vi "SaveDown.vi"(9 "DataPile":T1(array[cluster]), 10 "Analytes":string[](array[string])) -> ()   [LabVIEW 2024]
panel:
  in  "t0":timestamp
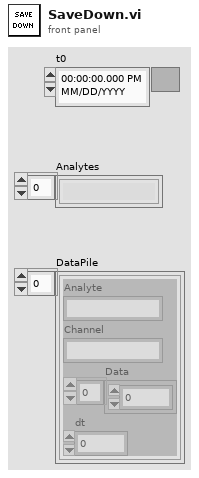
[diagram p1: front panel]
types:
  T1 = cluster{"Analyte":string, "Channel":string, "Data":dbl[], "dt":dbl}[]
  T2 = enum16{"open", "open or create", "create or replace", "create", "open (read-only)"}
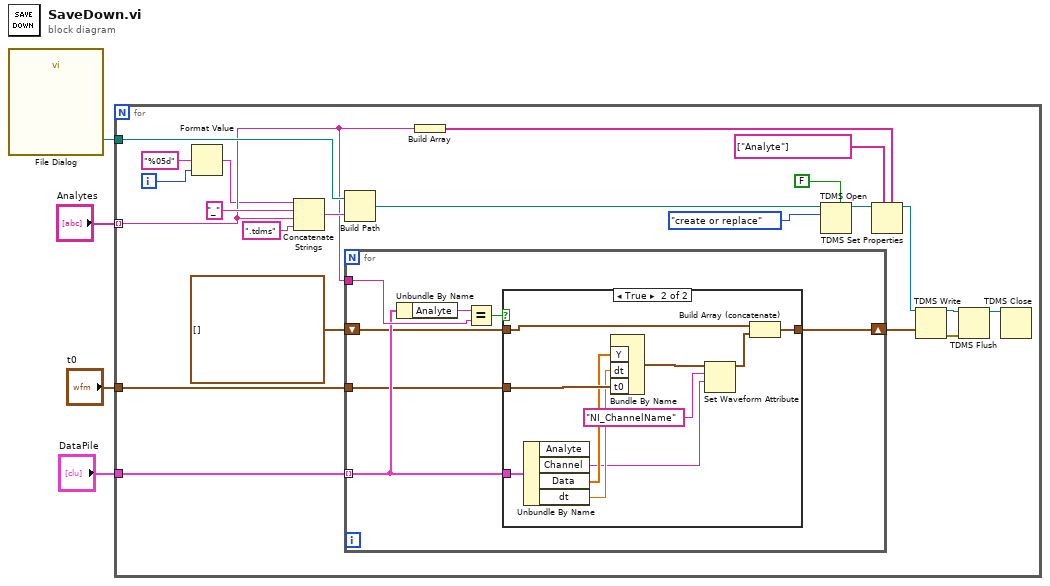
[diagram p0: block diagram]
diagram:
  n1 = call "File Dialog"() -> ("selected path"=w4:path)  [unwired: 12 in, 3 out]
  n2 = for {
    tunnel: "Analytes" -> [w13] mode=indexing
    tunnel: "DataPile" -> [w26]
    tunnel: "t0" -> [w25]
    tunnel: w4 -> [w22]
    i -> [w10]
    n3 = Format Value(format string="%05d", value (0)=w10) -> (output string=w8:string)  [unwired: 1 in]
    n4 = Concatenate Strings(w8, "_" ("string"), w13, ".tdms" ("string")) -> (w20:string)
    n5 = Build Path(base path=w22, name or relative path=w20) -> (appended path=w23:path)
    n6 = for {
      tunnel: w26 -> [w30] mode=indexing
      tunnel: w13 -> [w33]
      tunnel: w25 -> [w29]
      shift-right: [w27] -> w16
      shift-left: waveform(dbl)[] [] -> [w28]
      n7 = Unbundle By Name(w30) -> ("Analyte"=w32:string)
      n8 = Equal?(x=w32, y=w33) -> (x = y?=w31:bool)
      n9 = case shown="True" w31 {
        tunnel: w30 -> [_ w44]
        tunnel: w29 -> [_ w43]
        tunnel: w28 -> [w34 w36]
        tunnel: [w34 w35] -> w27
        frame False {
        }
        frame True {
          n10 = Unbundle By Name(w44) -> ("Channel"=w38:string, "Data"=w42:dbl[], "dt"=w41:dbl)  [unwired: 1 out]
          n11 = Bundle By Name("Y"=w42, "dt"=w41, "t0"=w43) -> (w40:waveform(dbl))  [unwired: 1 in]
          n12 = Set Waveform Attribute(5:w38, 6:"NI_ChannelName" ("name"), 7:w40) -> (3:w37:waveform(dbl))  [unwired: 1 in, 2 out]
          n13 = Build Array (concatenate)(w36, w37) -> (w35:waveform(dbl)[])
        }
      }
    }
    n14 = Build Array(w13) -> (w11:string[])
    n15 = TDMS Open(5:FALSE ("create index file? (T)"), 10:T2."create or replace" ("operation (0:open)"), 11:w23) -> (3:w18:refnum<k34>)  [unwired: 4 in, 1 out]
    n16 = TDMS Set Properties(5:w11, 7:string[] ["Analyte"], 11:w18) -> (3:w14:refnum<k34>)  [unwired: 3 in, 3 out]
    n17 = TDMS Write(0:w14, 9:w16) -> (4:w6:refnum<k34>, 15:w7:errorcluster)  [unwired: 4 in, 2 out]
    n18 = TDMS Flush(4:w7, 7:w6) -> (3:w5:refnum<k34>)  [unwired: 1 out]
    n19 = TDMS Close(11:w5) -> ()  [unwired: 1 in, 2 out]
  }
